vi "Measure.vi"(8 "error in (no error)":errorcluster, 9 "measurement configuration":variant, 10 "measure call context in":refnum<class "Measure Call Context.lvclass">, 11 "measurement plugin in":refnum<class "I2C Bus Monitor.lvclass">) -> (0 "error out":errorcluster, 1 "measurement results":variant, 2 "measure call context out":refnum<class "Measure Call Context.lvclass">, 3 "measurement plugin out":refnum<class "I2C Bus Monitor.lvclass">)   [LabVIEW 2025, in "I2C Bus Monitor.lvclass"]
uses:
  I2C Bus Monitor.lvclass
  <vilib>/Plug-In SDKs/Measurements/Measure Call Context/Measure Call Context.lvclass
  Measurement Configuration.ctl
  OOB gRPC Server/OOB gRPC Server.lvlib
  OOB Data Transfer/OOB Data Transfer.lvlib
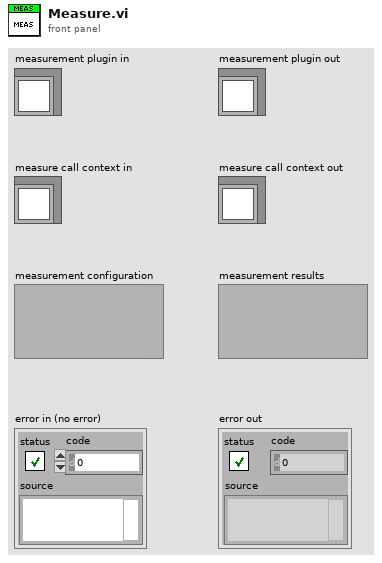
[diagram p1: front panel]
types:
  T1 = typedef "I2C Bus Monitor.lvclass/Measurement Configuration.ctl" = cluster{"Dummy":dbl}
  T2 = typedef "I2C Bus Monitor.lvclass/Measurement Results.ctl" = cluster{"OOB gRPC Port":i32, "PauseResume (Loopback)":bool, "Export (Loopback)":string, "Measurement Logic Counter":i32}
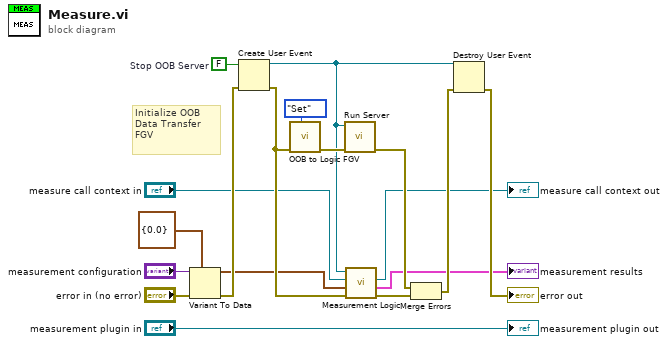
[diagram p0: block diagram]
diagram:
  w4 = FALSE  # Stop OOB Server
  # "Initialize OOB Data Transfer FGV"
  n1 = Variant To Data(error in="error in (no error)", type=T1 {"Dummy"=0.0} ("measurement configuration"), Variant="measurement configuration") -> (data=w5:T1, error out=w18:errorcluster)
  n2 = Create User Event(user event datatype=w4, error in=w18) -> (user event=w1:refnum<user-event>, error out=w17:errorcluster)
  n3 = call "OOB to Logic FGV.vi"("Op (Get)"=enum16{"Get", "Set"}."Set", "error in (no error)"=w17) -> ("error out"=w3:errorcluster)  [unwired: 8 in, 1 out]
  n4 = call "Run Server.vi"("error in (no error)"=w3, "Stop OOB Server UE"=w1) -> ("error out"=w16:errorcluster)  [unwired: 9 in]
  n5 = call "Measurement Logic.vi"("error in"=w17, "measurement configuration"=w5, "measure call context in"="measure call context in", "Stop OOB Server UE"=w1) -> ("error out"=w13:errorcluster, "measurement results"=→"measurement results":T2, "measure call context out"=→"measure call context out":refnum<class "Measure Call Context.lvclass">)  [unwired: 5 in]
  n6 = Merge Errors(w16, w13) -> (w15:errorcluster)
  n7 = Destroy User Event(user event=w1, error in=w15) -> (error out=→"error out":errorcluster)
  "measurement plugin out" <- "measurement plugin in"
